vi "Initialize Digital and Analog devices.vi"(8 "error in":errorcluster, 10 "Analog initialize settings":T2={"analog acquisition channel"="", "samples per channel"=1000, "sample rate"=1000.0} {"sample rate" format="%0.2f"}, 11 "Digital initialize settings":T3) -> (0 "error out":errorcluster, 2 "analog task":refnum<k21>, 3 "master clock task":T1, 5 "digital audio task":T1)   [LabVIEW 2021]
uses:
  controls/Digital Initialize Settings.ctl
  <vilib>/PDM Acquisition Toolkit/host/Classes/Tasks/I2S Output/Control/SignalProperties.ctl
  <vilib>/PDM Acquisition Toolkit/host/Classes/Channels/I2S Ouput/Controls/GenerationChannelProperties.ctl
  controls/Analog Initialize Settings.ctl
  <vilib>/PDM Acquisition Toolkit/host/Classes/Tasks/PCM Output/Controls/PCM Output Task DVR.ctl
  <vilib>/PDM Acquisition Toolkit/host/Classes/Tasks/PCM Output/PCM Output Task.lvclass
  <vilib>/PDM Acquisition Toolkit/shared/controls/clock mode.ctl
  <vilib>/PDM Acquisition Toolkit/shared/controls/PCM Data Format Configuration.ctl
  <vilib>/PDM Acquisition Toolkit/shared/controls/Digital Edge.ctl
  <vilib>/PDM Acquisition Toolkit/shared/controls/PCM Bit Endianness.ctl
  <vilib>/PDM Acquisition Toolkit/shared/controls/PCM Data Justification.ctl
  <vilib>/PDM Acquisition Toolkit/shared/controls/PCM Frame Sync Control.ctl
  <vilib>/PDM Acquisition Toolkit/host/Classes/Session/Controls/Logic Levels.ctl
  <vilib>/DAQmx/create/channels.llb/DAQmx Create Channel (AI-Voltage-Basic).vi
  <vilib>/DAQmx/configure/timing.llb/DAQmx Timing (Sample Clock).vi
  <vilib>/PDM Acquisition Toolkit/host/API/Public/Function Generator/Configure Custom Signal (N Ch) - PCM Output Task.vi
  digital audio protocol/digital audio protocol controls.lvlib
  <vilib>/PDM Acquisition Toolkit/host/API/PDM Acquisition Toolkit.lvlib
  <vilib>/PDM Acquisition Toolkit/shared/PDM Shared.lvlib
  <vilib>/PDM Acquisition Toolkit/host/Classes/Session/DecoderSession.lvclass
  <vilib>/PDM Acquisition Toolkit/host/Classes/Channels/I2S Ouput/I2S Output Channel.lvclass
  <vilib>/PDM Acquisition Toolkit/host/Classes/Tasks/I2S Output/I2S Output Task.lvclass
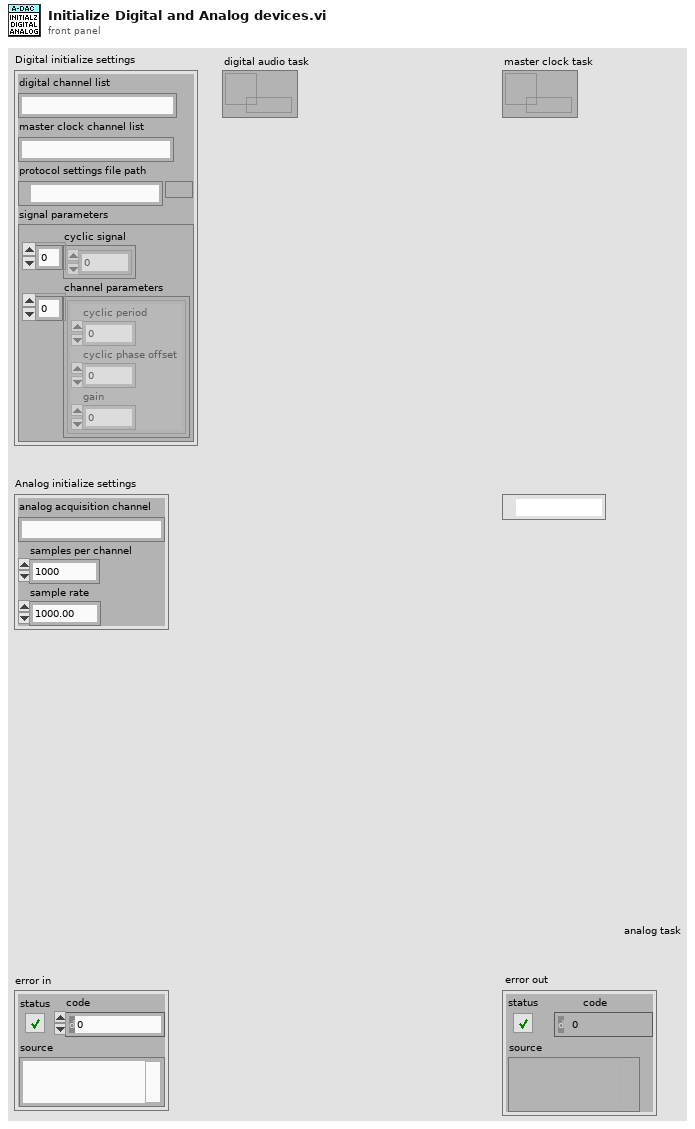
[diagram p1: front panel]
types:
  T1 = typedef "PDM Acquisition Class Library.lvlib/PCM Output Task.lvclass/PCM Output Task DVR.ctl" = refnum<data-value>
  T2 = typedef "Analog Initialize Settings.ctl" = cluster{"analog acquisition channel":string, "samples per channel":i32, "sample rate":dbl}
  T3 = typedef "Digital Initialize Settings.ctl" = cluster{"digital channel list":string, "master clock channel list":string, "protocol settings file path":path, "signal parameters":T4}
  T4 = typedef "PDM Acquisition Class Library.lvlib/I2S Output Task.lvclass/SignalProperties.ctl" = cluster{"cyclic signal":dbl[], "channel parameters":T5[]}
  T5 = typedef "PDM Acquisition Class Library.lvlib/I2S Output Channel.lvclass/GenerationChannelProperties.ctl" = cluster{"cyclic period":dbl, "cyclic phase offset":dbl, "gain":dbl}
  T6 = typedef "PDM Shared.lvlib/PCM Frame Sync Control.ctl" = cluster{"Frame Length":u16, "Frame Sync Pulse Width":u16, "Bit Clock Edge  Sync":T7}
  T7 = typedef "PDM Shared.lvlib/Digital Edge.ctl" = enum8{"Rising", "Falling"}
  T8 = typedef "PDM Shared.lvlib/PCM Data Format Configuration.ctl" = cluster{"Frame Sync Edge for Channel 0":T7, "Channel Count Per Frame":u8, "Channel Length":u16, "Bit Depth":u8, "Channel 0 Offset":u16, "Endianness":T9, "Data Justification":T10}
  T9 = typedef "PDM Shared.lvlib/PCM Bit Endianness.ctl" = enum16{"MSB First", "LSB First"}
  T10 = typedef "PDM Shared.lvlib/PCM Data Justification.ctl" = enum16{"Left Justified", "Right Justified"}
  T11 = typedef "PDM Shared.lvlib/clock mode.ctl" = enum16{"divided clock", "DDS"}
  T12 = typedef "digital audio protocol controls.lvlib/digital audio protocol settings.ctl" = cluster{"number of channels":u32, "data justification":string, "endianness":string, "channel length":u32, "bit depth":u32, "frame clock rate":dbl, "bit clock edge sync":string, "master clock rate":dbl, "logic level":string, "frame sync edge for channel 0":string, "Channel 0 Offset":u32}
  T13 = typedef "PDM Acquisition Class Library.lvlib/DecoderSession.lvclass/Logic Levels.ctl" = enum16{"3.3 V", "1.8 V", "1.2 V"}
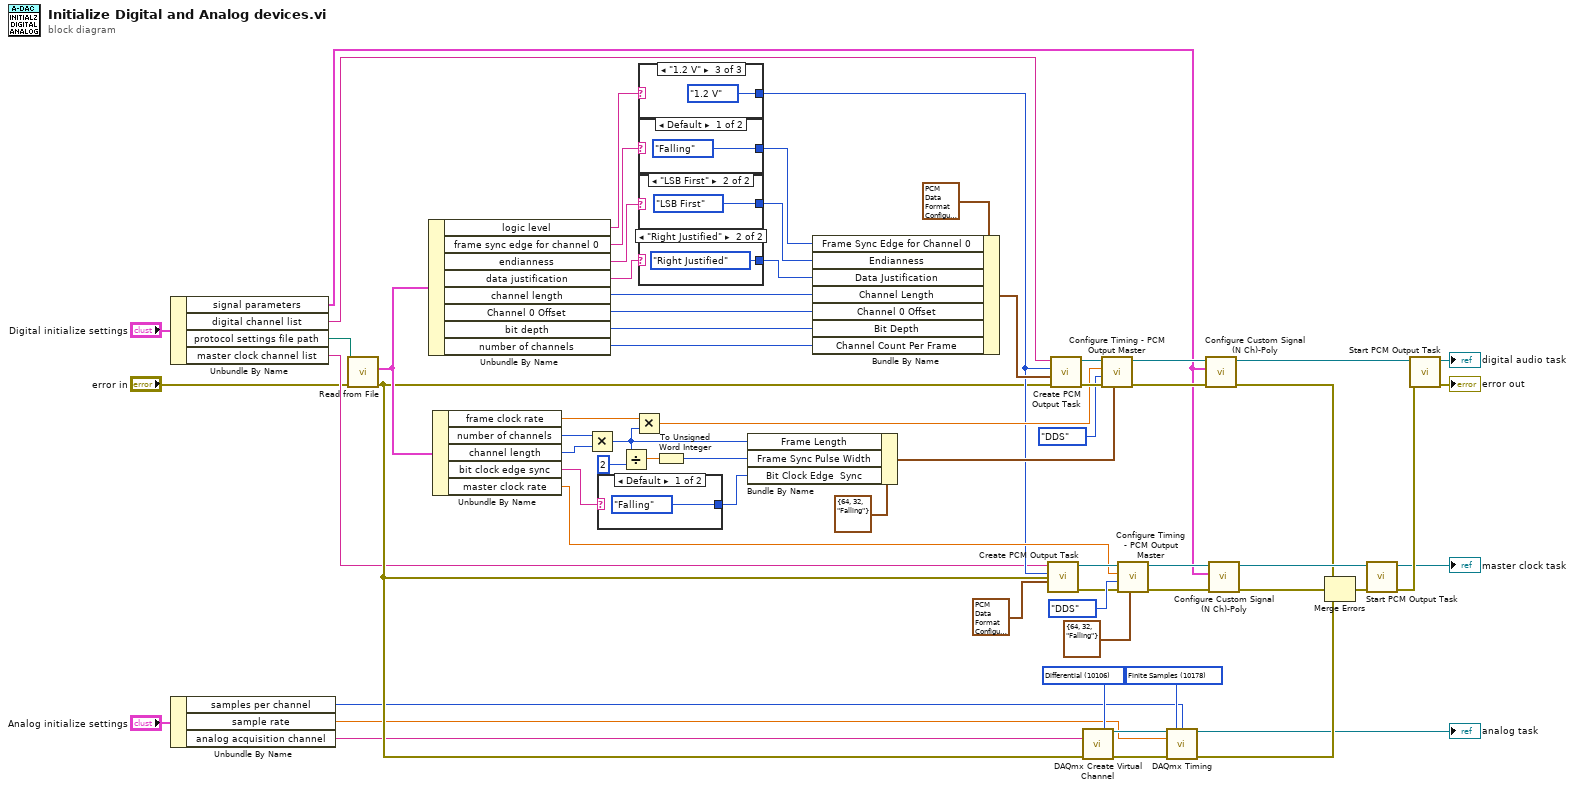
[diagram p0: block diagram]
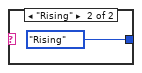
[diagram p2: hidden frame]
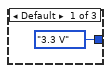
[diagram p3: hidden frame]
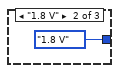
[diagram p4: hidden frame]
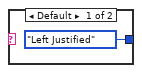
[diagram p5: hidden frame]
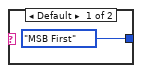
[diagram p6: hidden frame]
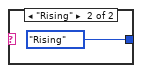
[diagram p7: hidden frame]
diagram:
  w23 = 10106 items=["Default"=-1, "RSE"=10083, "NRSE"=10078, "Differential"=10106, "Pseudodifferential"=12529] ("input terminal configuration")
  w24 = 10178 items=["Finite Samples"=10178, "Continuous Samples"=10123, "Hardware Timed Single Point"=12522] ("sample mode")
  n1 = Unbundle By Name("Digital initialize settings") -> ("signal parameters"=w10:T4, "digital channel list"=w11:string, "protocol settings file path"=w13:path, "master clock channel list"=w12:string)
  n2 = Unbundle By Name("Analog initialize settings") -> ("samples per channel"=w6:i32, "sample rate"=w7:dbl, "analog acquisition channel"=w8:string)
  n3 = call "Read from File.vi"("error in (no error)"="error in", "file path"=w13) -> ("error out"=w22:errorcluster, "digital audio protocol settings"=w41:T12)  [unwired: 7 in, 1 out]
  n4 = Unbundle By Name(w41) -> ("logic level"=w56:string, "frame sync edge for channel 0"=w62:string, "endianness"=w60:string, "data justification"=w58:string, "channel length"=w63:u32, "Channel 0 Offset"=w64:u32, "bit depth"=w65:u32, "number of channels"=w66:u32)
  n5 = Unbundle By Name(w41) -> ("frame clock rate"=w42:dbl, "number of channels"=w50:u32, "channel length"=w49:u32, "bit clock edge sync"=w45:string, "master clock rate"=w32:dbl)
  n6 = Multiply(x=w50, y=w49) -> (x*y=w43:u32)
  n7 = case shown="Default" w45 {
    tunnel: [Digital_Edge."Falling" ("Frame Sync Edge for Channel 0") Digital_Edge."Rising" ("Frame Sync Edge for Channel 0")] -> w44
    frame Default {
    }
    frame "Rising" {
    }
  }
  n8 = Divide(x=w43, y=u32 2) -> (x/y=w47:dbl)
  n9 = Multiply(x=w42, y=w43) -> (x*y=w40:dbl)
  n10 = case shown="\"1.2 V\"" w56 {
    tunnel: [Logic_Levels."3.3 V" ("logic level") Logic_Levels."1.8 V" ("logic level") Logic_Levels."1.2 V" ("logic level")] -> w31
    frame Default {
    }
    frame "1.8 V" {
    }
    frame "1.2 V" {
    }
  }
  n11 = case shown="Default" w62 {
    tunnel: [Digital_Edge."Falling" ("Frame Sync Edge for Channel 0") Digital_Edge."Rising" ("Frame Sync Edge for Channel 0")] -> w61
    frame Default {
    }
    frame "Rising" {
    }
  }
  n12 = case shown="\"LSB First\"" w60 {
    tunnel: [PCM_Bit_Endianness."MSB First" ("Endianness") PCM_Bit_Endianness."LSB First" ("Endianness")] -> w59
    frame Default {
    }
    frame "LSB First" {
    }
  }
  n13 = case shown="\"Right Justified\"" w58 {
    tunnel: [PCM_Data_Justification."Left Justified" ("Data Justification") PCM_Data_Justification."Right Justified" ("Data Justification")] -> w57
    frame Default {
    }
    frame "Right Justified" {
    }
  }
  n14 = To Unsigned Word Integer(number=w47) -> (unsigned 16bit integer=w46:u16)
  n15 = Bundle By Name(cluster=T6 {"Frame Length"=64, "Frame Sync Pulse Width"=32, "Bit Clock Edge  Sync"=enum."Falling"} ("Frame Sync Clock Control"), "Frame Length"=w43, "Frame Sync Pulse Width"=w46, "Bit Clock Edge  Sync"=w44) -> (w39:T6)
  n16 = Bundle By Name(cluster=T8 {"Frame Sync Edge for Channel 0"=enum."Falling", "Channel Count Per Frame"=2, "Channel Length"=32, "Bit Depth"=24, "Channel 0 Offset"=1, "Endianness"=enum."MSB First", "Data Justification"=enum."Left Justified"} ("PCM data configuration"), "Frame Sync Edge for Channel 0"=w61, "Endianness"=w59, "Data Justification"=w57, "Channel Length"=w63, "Channel 0 Offset"=w64, "Bit Depth"=w65, "Channel Count Per Frame"=w66) -> (w54:T8)
  n17 = call <vilib>:"Create PCM Output Task.vi"("error in"=w22, "PCM data configuration"=T8 {"Frame Sync Edge for Channel 0"=enum."Falling", "Channel Count Per Frame"=2, "Channel Length"=32, "Bit Depth"=24, "Channel 0 Offset"=1, "Endianness"=enum."MSB First", "Data Justification"=enum."Left Justified"}, "logic level"=w31, "channel list"=w12) -> ("error out"=w36:errorcluster, "PCM output task out"=w35:T1)  [unwired: 6 in]
  n18 = call <vilib>:"Create PCM Output Task.vi"("error in"=w22, "PCM data configuration"=w54, "logic level"=w31, "channel list"=w11) -> ("error out"=w52:errorcluster, "PCM output task out"=w53:T1)  [unwired: 6 in]
  n19 = call-poly <vilib>:"DAQmx Create Virtual Channel.vi"("input terminal configuration"=w23, "physical channels"=w8, "error in"=w22) -> ("task out"=w25:refnum<k21>, "error out"=w26:errorcluster)  [unwired: 11 in]
  n20 = call <vilib>:"Configure Timing - PCM Output Master.vi"("Frame Sync Clock Control"=w39, "error in"=w52, "clock mode"=clock_mode."DDS", "Bit Clock rate"=w40, "PCM output task in"=w53) -> ("error out"=w29:errorcluster, "PCM output task out"=w30:T1)  [unwired: 4 in, 1 out]
  n21 = call <vilib>:"Configure Timing - PCM Output Master.vi"("Frame Sync Clock Control"=T6 {"Frame Length"=64, "Frame Sync Pulse Width"=32, "Bit Clock Edge  Sync"=enum."Falling"}, "error in"=w36, "clock mode"=clock_mode."DDS", "Bit Clock rate"=w32, "PCM output task in"=w35) -> ("error out"=w27:errorcluster, "PCM output task out"=w28:T1)  [unwired: 4 in, 1 out]
  n22 = call-poly <vilib>:"DAQmx Timing.vi"("task/channels in"=w25, "sample mode"=w24, "samples per channel"=w6, "rate"=w7, "error in"=w26) -> ("task out"=→"analog task":refnum<k21>, "error out"=w15:errorcluster)  [unwired: 9 in]
  n23 = call-poly <vilib>:"Configure Custom Signal (N Ch)-Poly.vi"("error in"=w29, "signal parameters"=w10, "PCM output task in"=w30) -> ("error out"=w17:errorcluster, "PCM output task out"=w18:T1)  [unwired: 7 in]
  n24 = call-poly <vilib>:"Configure Custom Signal (N Ch)-Poly.vi"("error in"=w27, "signal parameters"=w10, "PCM output task in"=w28) -> ("error out"=w16:errorcluster, "PCM output task out"=w19:T1)  [unwired: 7 in]
  n25 = Merge Errors(w17, w16, w15) -> (w20:errorcluster)
  n26 = call <vilib>:"Start PCM Output Task.vi"("error in"=w20, "PCM output task in"=w19) -> ("error out"=w21:errorcluster, "PCM output task out"=→"master clock task":T1)  [unwired: 8 in]
  n27 = call <vilib>:"Start PCM Output Task.vi"("error in"=w21, "PCM output task in"=w18) -> ("error out"=→"error out":errorcluster, "PCM output task out"=→"digital audio task":T1)  [unwired: 8 in]
